vi "Create Thing.vi"(6 "Attributes":T1[](array[typedef]), 8 "error in (no error)":errorcluster, 9 "Type":string, 10 "Name":string, 11 "IoT Session in":refnum<class "IoT Session.lvclass">) -> (0 "error out":errorcluster, 3 "IoT Session out":refnum<class "IoT Session.lvclass">)   [LabVIEW 2015, in "NI_AWS_IoT.lvlib" / "IoT Session.lvclass"]
uses:
  IoT Session.lvclass
  Core/HTTP Request/Name Value Pair.ctl
  Core/HTTP Request/Valid String Specification.ctl
  Core/HTTP Request/Request Options.ctl
  Core/HTTP Request/Region handling.ctl
  Core/HTTP Request/URL formatting.ctl
  Core/HTTP Request/HTTP Request.lvclass
  NI_AWS_IoT.lvlib
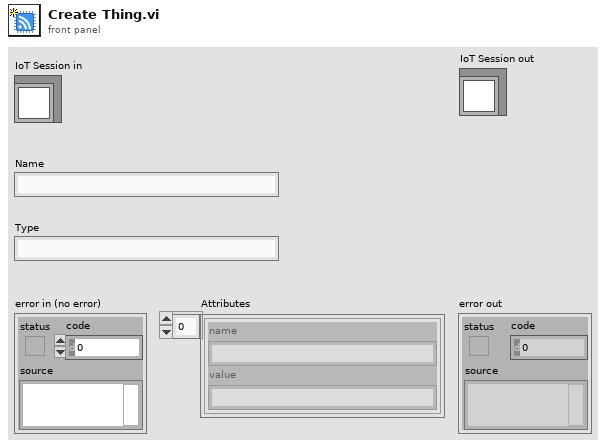
[diagram p1: front panel]
types:
  T1 = typedef "NI_AWS_Core.lvlib/HTTP Request.lvclass/Name Value Pair.ctl" = cluster{"name":string, "value":string}
  T2 = typedef "NI_AWS_Core.lvlib/HTTP Request.lvclass/Valid String Specification.ctl" = enum16{"none", "only [alphanumeric][-][_]", "only [alphanumeric][-][_][space]", "phone number +1xxxyyyzzzz", "Regular Expression"}
  T3 = typedef "NI_AWS_Core.lvlib/HTTP Request.lvclass/Request Options.ctl" = cluster{"request headers":T1[], "request parameters":T1[], "request body":string, "region handling":T4, "URL formatting":T5}
  T4 = typedef "NI_AWS_Core.lvlib/HTTP Request.lvclass/Region handling.ctl" = enum16{"use region everywhere", "use region (authentication only)", "use region (URL only)", "ignore region everwhere"}
  T5 = typedef "NI_AWS_Core.lvlib/HTTP Request.lvclass/URL formatting.ctl" = enum16{"region-", "region."}
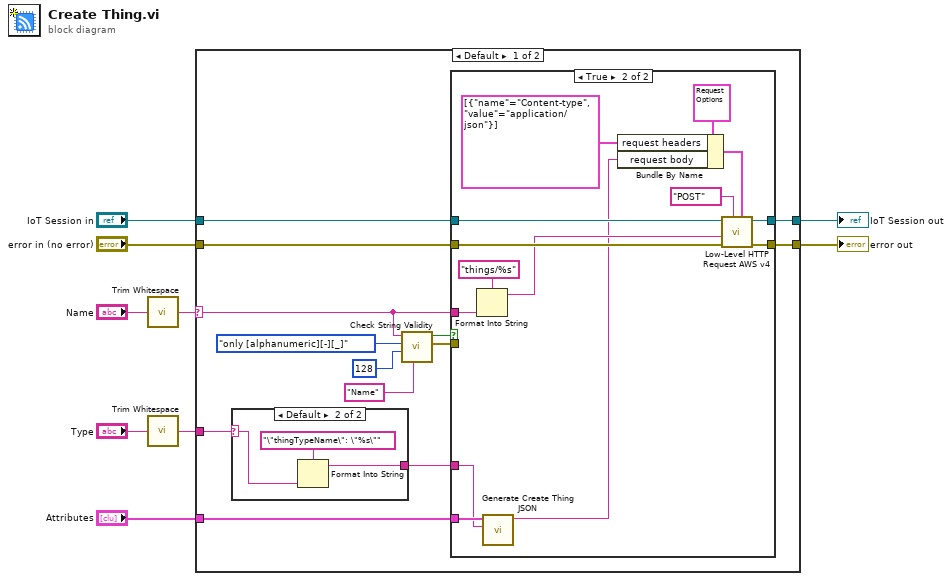
[diagram p0: block diagram]
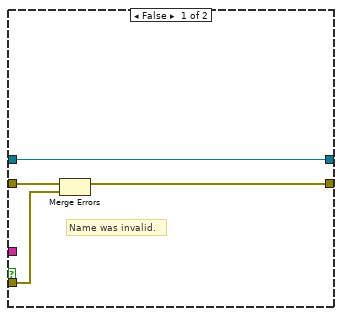
[diagram p2: hidden frame]
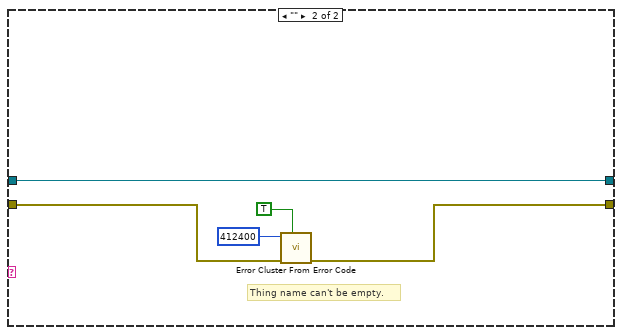
[diagram p4: hidden frame]
diagram:
  n1 = call <vilib>:"Trim Whitespace.vi"("string"="Name") -> ("trimmed string"=w5:string)  [unwired: 1 in]
  n2 = call <vilib>:"Trim Whitespace.vi"("string"="Type") -> ("trimmed string"=w3:string)  [unwired: 1 in]
  n3 = case shown="Default" w5 {
    selector: w5 -> [w15 _]
    tunnel: "error in (no error)" -> [w22 w48]
    tunnel: [w21 w47] -> w8
    tunnel: [w20 w45] -> w7
    tunnel: w3 -> [w14 _]
    tunnel: "IoT Session in" -> [w12 w45]
    tunnel: "Attributes" -> [w10 _]
    frame Default {
      n4 = case shown="Default" w14 {
        selector: w14 -> [_ w42]
        tunnel: [_ w41] -> w11
        frame "" {
        }
        frame Default {
          n5 = Format Into String(format string="\"thingTypeName\": \"%s\"", w42) -> (resulting string=w41:string)  [unwired: 2 in, 1 out]
        }
      }
      n6 = call "Check String Validity.vi"("String Name for Error"="Name", "Max Characters"=128, "Valid String Specification"=Valid_String_Specification."only [alphanumeric][-][_]", "String"=w15) -> ("string error"=w16:errorcluster, "Valid"=w13:bool)  [unwired: 6 in]
      n7 = case shown="True" w13 {
        tunnel: w22 -> [w26 w40]
        tunnel: [w25 w39] -> w21
        tunnel: [w23 w38] -> w20
        tunnel: w15 -> [_ w34]
        tunnel: w16 -> [w24 _]
        tunnel: w12 -> [w23 w30]
        tunnel: w11 -> [_ w28]
        tunnel: w10 -> [_ w29]
        frame False {
          # "Name was invalid."
          n8 = Merge Errors(w26, w24) -> (w25:errorcluster)
        }
        frame True {
          n9 = Format Into String(format string="things/%s", w34) -> (resulting string=w35:string)  [unwired: 2 in, 1 out]
          n10 = call "Generate Create Thing JSON.vi"("Thing Type JSON"=w28, "Attributes"=w29) -> ("Create Thing JSON"=w27:string)  [unwired: 9 in]
          n11 = Bundle By Name(cluster=T3 {"request headers"=[], "request parameters"=[], "request body"="", "region handling"=enum."use region everywhere", "URL formatting"=enum."region."} ("Request Options"), "request headers"=T1[] [{"name"="Content-type", "value"="application/json"}], "request body"=w27) -> (w32:T3)
          n12 = call "Low-Level HTTP Request AWS v4.vi"("Request Options"=w32, "HTTP-Verb"="POST", "error in (no error)"=w40, "URL Suffix"=w35, "AWS Core in"=w30) -> ("error out"=w39:errorcluster, "AWS Core out"=w38:refnum<class "IoT Session.lvclass">)  [unwired: 3 in, 2 out]
        }
      }
    }
    frame "" {
      # "Thing name can't be empty."
      n13 = call <vilib>:"Error Cluster From Error Code.vi"("show call chain? (False)"=TRUE, "error in (no error)"=w48, "error code (0)"=412400) -> ("error out"=w47:errorcluster)  [unwired: 6 in]
    }
  }
  "error out" <- w8
  "IoT Session out" <- w7
